vi "Write Misc Settings.vi"(4 "Section":string, 5 "error in (no error)":errorcluster, 6 "p_value":string, 7 "Key":string, 8 "Config Data_DB_ADO in":refnum<class "Config Data_DB_ADO.lvclass">) -> (0 "error out":errorcluster, 3 "Config Data_DB_ADO out":refnum<class "Config Data_DB_ADO.lvclass">)   [LabVIEW 2020, in "Config Data.lvlib" / "Config Data_DB_ADO.lvclass"]
uses:
  Config Data_DB_ADO.lvclass
  toolbox/ADO Database Drivers/ADO Database Drivers.lvlib
  Config Data_DB.lvclass
  C:/Users/Fred Guo/Desktop/Release 19/_libraries/Config Data/DB/Config Data_DB.lvclass
  C:/Users/Fred Guo/Desktop/Release 19/_libraries/Config Data/Config Data.lvclass
  C:/Users/Fred Guo/Desktop/Release 19/_libraries/Config Data/DB/ADO/Config Data_DB_ADO.lvclass
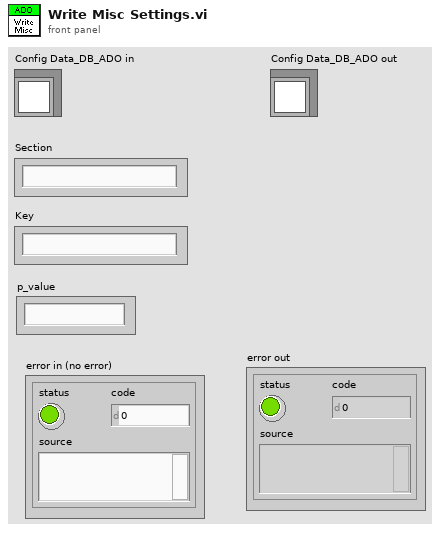
[diagram p1: front panel]
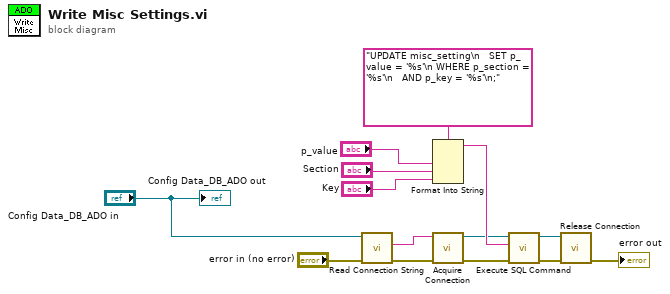
[diagram p0: block diagram]
diagram:
  n1 = call "Read Connection String.vi"("Error In"="error in (no error)", "DB In"="Config Data_DB_ADO in") -> ("Error Out"=w9:errorcluster, "Connection String"=w14:string)  [unwired: 3 in, 1 out]
  n2 = Format Into String(format string="UPDATE misc_setting\n   SET p_value = '%s'\n WHERE p_section = '%s'\n   AND p_key = '%s'\n;", "p_value", "Section", "Key") -> (resulting string=w11:string)  [unwired: 2 in, 1 out]
  n3 = call "Acquire Connection.vi"("error in (no error)"=w9, "Connection String"=w14) -> ("error out"=w7:errorcluster, "Connection"=w8:refnum<k7>)  [unwired: 3 in, 1 out]
  n4 = call "Execute SQL Command.vi"("error in"=w7, "SQL Command"=w11, "Connection In"=w8) -> ("error out"=w13:errorcluster, "Connection Out"=w12:refnum<k7>)  [unwired: 2 in, 1 out]
  n5 = call "Release Connection.vi"("error in"=w13, "Connection"=w12) -> ("error out"=→"error out":errorcluster)  [unwired: 5 in]
  "Config Data_DB_ADO out" <- "Config Data_DB_ADO in"
